vi "Save 1D Trace (cpx).vi"(4 "Data Type":T2(ring)=enum."complex64", 6 "Contents ID":string="TRACE", 8 "Error In":errorcluster, 9 "Trace":T1 {"Z" format="%#_4g"}, 11 "File Path":path) -> (0 "Error Out":errorcluster, 3 "File Refnum Out":refnum<file>)   [LabVIEW 2016]
uses:
  Processing/Trace (cplx).ctl
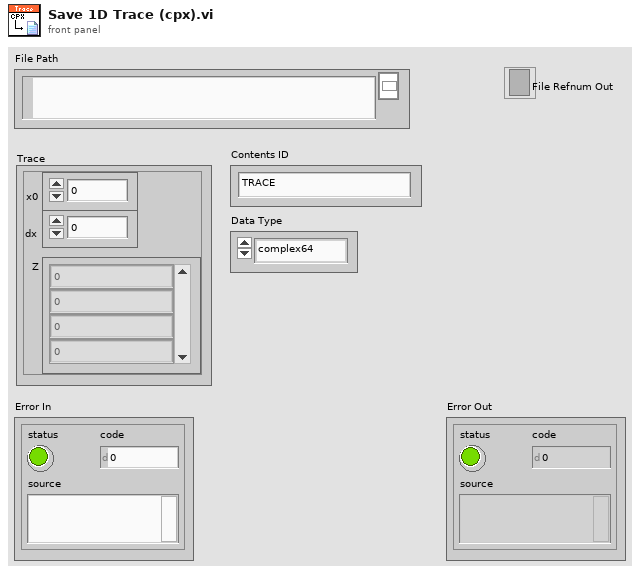
[diagram p1: front panel]
types:
  T1 = typedef "Trace (cplx).ctl" = cluster{"x0":dbl, "dx":dbl, "Z":cdb[]}
  T2 = enum16{"int8", "int16", "int32", "uint8", "uint16", "uint32", "float32", "float64", "complex64", "complex128"}
  T3 = enum16{"open", "replace", "create", "open or create", "replace or create", "replace or create with confirmation"}
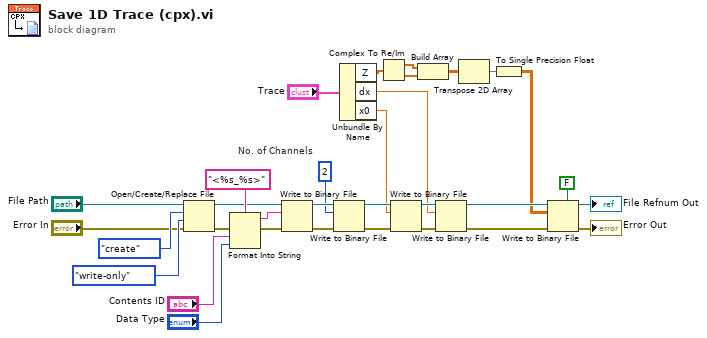
[diagram p0: block diagram]
diagram:
  w18 = 2  # No. of Channels
  n1 = Open/Create/Replace File(file path (use dialog)="File Path", error in="Error In", operation (0:open)=T3."create", access (0:read/write)=enum16{"read/write", "read-only", "write-only"}."write-only") -> (refnum out=w16:refnum<file>, error out=w17:errorcluster)  [unwired: 2 in, 1 out]
  n2 = Format Into String(format string="<%s_%s>", error in=w17, "Contents ID", "Data Type") -> (resulting string=w20:string, error out=w27:errorcluster)  [unwired: 1 in]
  n3 = Write to Binary File(file (use dialog)=w16, data=w20, error in=w27) -> (refnum out=w22:refnum<file>, error out=w21:errorcluster)  [unwired: 3 in, 1 out]
  n4 = Write to Binary File(file (use dialog)=w22, data=w18, error in=w21) -> (refnum out=w23:refnum<file>, error out=w25:errorcluster)  [unwired: 3 in, 1 out]
  n5 = Unbundle By Name("Trace") -> ("Z"=w9:cdb[], "dx"=w11:dbl, "x0"=w12:dbl)
  n6 = Complex To Re/Im(x + iy=w9) -> (x=w2:dbl[], y=w1:dbl[])
  n7 = Write to Binary File(file (use dialog)=w23, data=w12, error in=w25) -> (refnum out=w24:refnum<file>, error out=w26:errorcluster)  [unwired: 3 in, 1 out]
  n8 = Build Array(w2, w1) -> (w10:dbl[][])
  n9 = Write to Binary File(file (use dialog)=w24, data=w11, error in=w26) -> (refnum out=w14:refnum<file>, error out=w13:errorcluster)  [unwired: 3 in, 1 out]
  n10 = Transpose 2D Array(2D array=w10) -> (transposed array=w4:dbl[][])
  n11 = To Single Precision Float(number=w4) -> (single precision float=w3:sgl[][])
  n12 = Write to Binary File(file (use dialog)=w14, data=w3, error in=w13, 5:FALSE ("prepend array or string size? (T)")) -> (refnum out=→"File Refnum Out":refnum<file>, error out=→"Error Out":errorcluster)  [unwired: 2 in, 1 out]
